vi "Find All Acyclic Frames.vi"(8 "error in":errorcluster, 11 "port":T1 format="%.0x") -> (0 "error out":errorcluster, 1 "acyclic frames":T2[](array[typedef]), 2 "acyclic frame triggers":T1[](array[typedef]) format="%.0x", 3 "port out":T1 format="%.0x")   [LabVIEW 2020, in "AIM MIL-STD-1553 Scripting.lvlib"]
doc: "Returns all of the <b>acyclic frames</b> in the specified <b>port</b>."
uses:
  AIM MIL-STD-1553 Scripting.lvlib
  <vilib>/NI VeriStand/Custom Device API/Custom Device Item Ref.ctl
  Shared/Acyclic Frame Definition.ctl
  <vilib>/NI VeriStand/Custom Device API/Custom Device API.lvlib
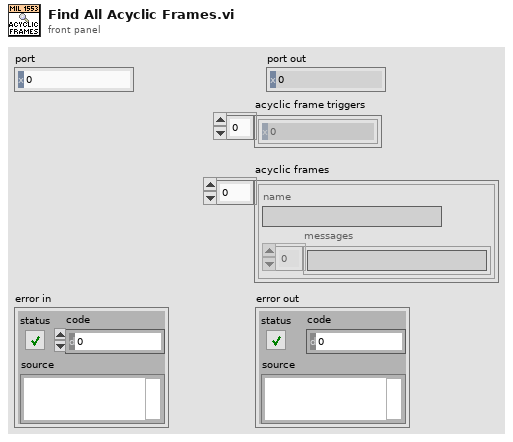
[diagram p1: front panel]
types:
  T1 = typedef "Custom Device API.lvlib/Custom Device Item Ref.ctl" = u64
  T2 = typedef "Acyclic Frame Definition.ctl" = cluster{"name":string, "messages":string[]}
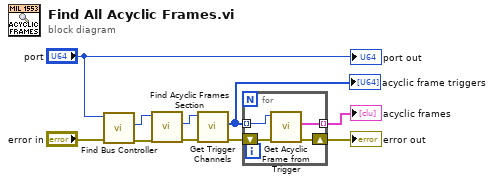
[diagram p0: block diagram]
diagram:
  n1 = call "Find Bus Controller.vi"("error in"="error in", "port"="port") -> ("error out"=w3:errorcluster, "bus controller"=w2:T1)  [unwired: 6 in, 2 out]
  n2 = call "Find Acyclic Frames Section.vi"("error in"=w3, "bus controller"=w2) -> ("error out"=w8:errorcluster, "acyclic frames section"=w9:T1)  [unwired: 6 in, 2 out]
  n3 = call "Get Trigger Channels.vi"("error in"=w8, "acyclic frames section"=w9) -> ("error out"=w7:errorcluster, "acyclic frame triggers"=w10:T1[])  [unwired: 6 in, 2 out]
  "acyclic frame triggers" <- w10
  n4 = for {
    tunnel: w10 -> [w14] mode=indexing
    shift-right: [w12] -> w6
    shift-left: w7 -> [w13]
    tunnel: [w11] -> w5 mode=indexing
    n5 = call "Get Acyclic Frame from Trigger.vi"("error in"=w13, "acyclic frame trigger"=w14) -> ("error out"=w12:errorcluster, "acyclic frame out"=w11:T2)  [unwired: 6 in, 2 out]
  }
  "error out" <- w6
  "acyclic frames" <- w5
  "port out" <- "port"
